vi "Link Subscriber Channel.vi"(8 "error in (no error)":errorcluster, 10 "Connection":T1, 11 "CIF_UI in":refnum<class "CIF_UI.lvclass">) -> (0 "error out":errorcluster)   [LabVIEW 2021, in "CIF_UI.lvclass"]
uses:
  CIF_UI.lvclass
  CIFCore/Grpc/CIFCoreChannel_client/RPC Messages/cif_channelcore_ConnectSubscriber.ctl
  CIF_UI.lvclass/CIF_UI.ctl
  CIFCore/Common/Typedef/Errors.ctl
  <vilib>/CIF Foundation/CIF Utilities/Errors/Append Error Location.vi
  CIFCore/Grpc/CIFCoreWrapper/CIFCoreWrapper.lvlib
  CIFCore/Common/CIFCoreCommon.lvlib
  CIFCore/Grpc/CIFCoreChannel_client/CIFCoreChannel_client.lvlib
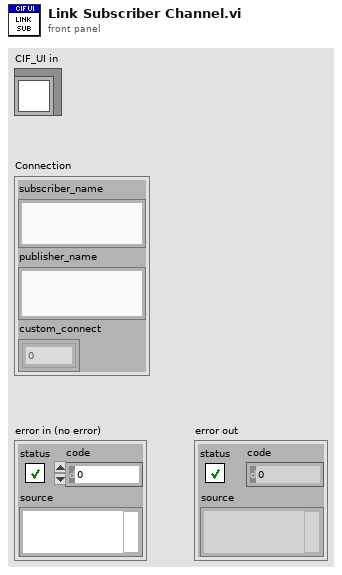
[diagram p1: front panel]
types:
  T1 = typedef "CIFCoreChannel_client.lvlib/cif_channelcore_ConnectSubscriber.ctl" = cluster{"subscriber_name":string, "publisher_name":string, "custom_connect":u8[]}
  T2 = typedef "CIF_UI.lvclass/Plugin Connection Map.ctl" = map{string, T3}
  T3 = typedef "CIF_UI.lvclass/Plugin Connections.ctl" = cluster{"gRPC ID":T4, "Plugin Info":T5}
  T4 = typedef "grpc-lvsupport-release.lvlib/grpcId.ctl" = u64
  T5 = typedef "CIF_UI.lvclass/PluginInfo.ctl" = cluster{"Name":string, "Type":string, "grpc_port":i32, "Version":T6, "Node Status":T7}
  T6 = typedef "CIF_UI.lvclass/Version.ctl" = cluster{"Major":i32, "Minor":i32, "Fix":i32}
  T7 = typedef "CIFCoreCommon.lvlib/gRPC Reported Plugin Status.ctl" = cluster{"State":T8, "Timing Statistics (us)":T9, "FIFO Statistics (us)":T11, "error":T12, "Monitor Doubles":T13, "Monitor U64":T14, "Monitor I64":T15}
  T8 = typedef "CIFCoreCommon.lvlib/Plugin State.ctl" = enum32{"Null", "Creating", "Listening", "Running", "CleaningUp", "Destroying"}
  T9 = typedef "CIFCoreCommon.lvlib/Timing Statistics.ctl" = cluster{"Period":T10, "Wake Error":T10, "Execute":T10, "Housekeep":T10, "Idle":T10, "Cleanup":T10, "Custom 1 (custom units)":T10, "Custom 2 (custom units)":T10}
  T10 = typedef "CIFCoreCommon.lvlib/Timing Stats Base.ctl" = cluster{"Max":i64, "Avg":dbl, "Min":i64}
  T11 = typedef "CIFCoreCommon.lvlib/FIFO Statistics.ctl" = cluster{"From T0":T10, "From Previous Plugin":T10, "Output Error":T10}
  T12 = typedef "CIFCoreCommon.lvlib/Simple Error.ctl" = cluster{"status":bool, "code":i32}
  T13 = typedef "CIFCoreCommon.lvlib/Monitor Doubles.ctl" = cluster{"1":dbl, "2":dbl, "3":dbl, "4":dbl}
  T14 = typedef "CIFCoreCommon.lvlib/Monitor U64.ctl" = cluster{"1":u64, "2":u64, "3":u64, "4":u64}
  T15 = typedef "CIFCoreCommon.lvlib/Monitor I64.ctl" = cluster{"1":i64, "2":i64, "3":i64, "4":i64}
  T16 = typedef "CIFCoreCommon.lvlib/Errors.ctl" = enum16{"Invalid Clock ID", "Long Sleep", "gRPC Server Not Found", "Config Parse", "Timestamp Wrap", "Delayed Execution", "Duplicate Channel", "Missing Channel", "Incorrect Type", "Flatten Error", "Unflatten Data", "Unique Name", "Plugin Not Found", "Plugin Type Not Found", "Plugin Version Not Found", "Manager Not Found", "Numerical Issue", "Time Jump", "Clock ID Match", "Channel Length", "Plugin Connection", "gRPC Server Connection", "PPL Name Match", "Build", "Config Log Parse", "Plugin Load", "UI Subpanel Load", "Python Name", "Invalid Name"}
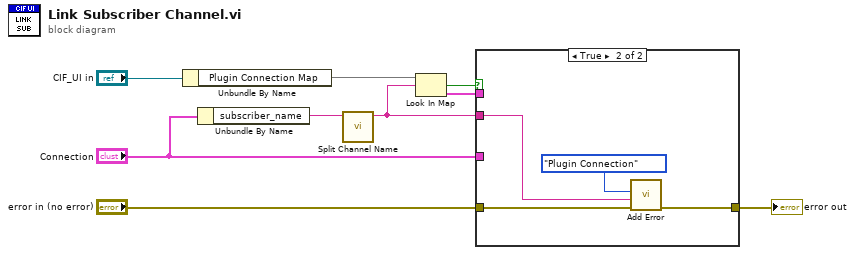
[diagram p0: block diagram]
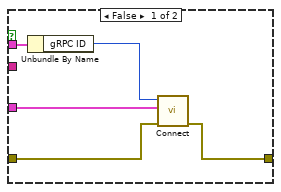
[diagram p2: hidden frame]
diagram:
  n1 = Unbundle By Name("CIF_UI in") -> ("Plugin Connection Map"=w9:T2)
  n2 = Unbundle By Name("Connection") -> ("subscriber_name"=w2:string)
  n3 = call "Split Channel Name.vi"("Channel Name"=w2) -> ("Parent"=w1:string)  [unwired: 8 in, 2 out]
  n4 = Look In Map(map=w9, key=w1) -> (key not found?=w7:bool, value=w6:T3)  [unwired: 1 in]
  n5 = case shown="True" w7 {
    tunnel: "error in (no error)" -> [w12 w17]
    tunnel: w6 -> [w14 _]
    tunnel: [w11 w16] -> w8
    tunnel: w1 -> [_ w15]
    tunnel: "Connection" -> [w10 _]
    frame False {
      n6 = Unbundle By Name(w14) -> ("gRPC ID"=w13:T4)
      n7 = call "Connect.vi"("error in"=w12, "Connection"=w10, "gRPC ID"=w13) -> ("error out"=w11:errorcluster)  [unwired: 7 in, 1 out]
    }
    frame True {
      n8 = call "Add Error.vi"("error in (no error)"=w17, "String to Append"=w15, "Error"=Errors."Plugin Connection") -> ("error out"=w16:errorcluster)  [unwired: 8 in]
    }
  }
  "error out" <- w8
